vi "Request Data JSON.vi"(8 "error in (no error)":errorcluster, 11 "SetInputMute in":refnum<class "SetInputMute.lvclass">) -> (0 "error out":errorcluster, 2 "Request Data JSON":string, 3 "SetInputMute out":refnum<class "SetInputMute.lvclass">)   [LabVIEW 2022 SP3, in "obs-websocket-lv.lvlib" / "SetInputMute.lvclass"]
uses:
  SetInputMute.lvclass
  SetInputMute.lvclass/SetInputMute.ctl
  <vilib>/IlluminatedG/lv-web-crypto/lv-json/JSON/JSON.lvlib
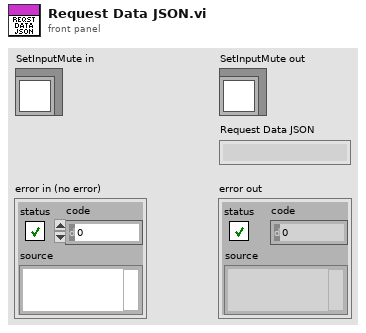
[diagram p1: front panel]
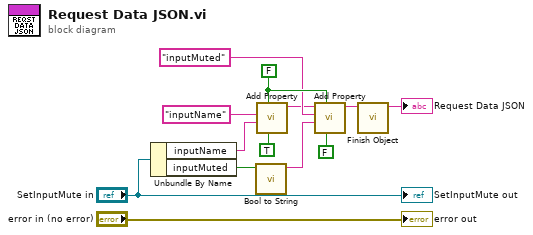
[diagram p0: block diagram]
diagram:
  w7 = FALSE ("Include Empty?")
  n1 = Unbundle By Name("SetInputMute in") -> ("inputName"=w11:string, "inputMuted"=w3:bool)
  n2 = call <vilib>:"Bool to String.vi"("Boolean"=w3) -> ("Value"=w2:string)  [unwired: 10 in]
  n3 = call <vilib>:"Add Property.vi"("String?"=TRUE, "Include Empty?"=w7, "Value"=w11, "Property Name"="inputName") -> ("String out"=w5:string)  [unwired: 7 in]
  n4 = call <vilib>:"Add Property.vi"("String?"=FALSE, "Include Empty?"=w7, "Value"=w2, "Property Name"="inputMuted", "String In"=w5) -> ("String out"=w4:string)  [unwired: 6 in]
  n5 = call <vilib>:"Finish Object.vi"("String In"=w4) -> ("String out"=→"Request Data JSON":string)  [unwired: 10 in]
  "error out" <- "error in (no error)"
  "SetInputMute out" <- "SetInputMute in"
